vi "Request Live Measurement.vi"(0 "Gas In":refnum<class "Gas.lvclass">, 5 "Request Type":u8=160 format="%x", 11 "error in (no error)":errorcluster) -> (4 "Gas Out":refnum<class "Gas.lvclass">, 6 "Success?":bool, 15 "error out":errorcluster)   [LabVIEW 2015, in "Gas.lvclass"]
uses:
  Gas.lvclass
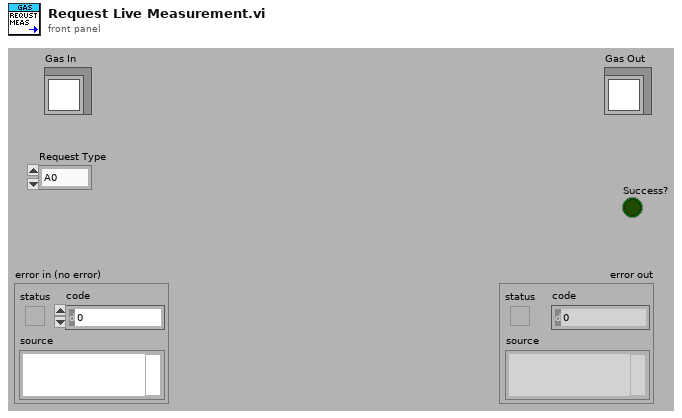
[diagram p1: front panel]
types:
  T1 = typedef "XNET Frame CAN.ctl" = cluster{"timestamp":timestamp, "payload":u8[], "identifier":u32, "type":T2, "extended?":bool, "echo?":bool}
  T2 = typedef "XNET Frame Type CAN.ctl" = u8
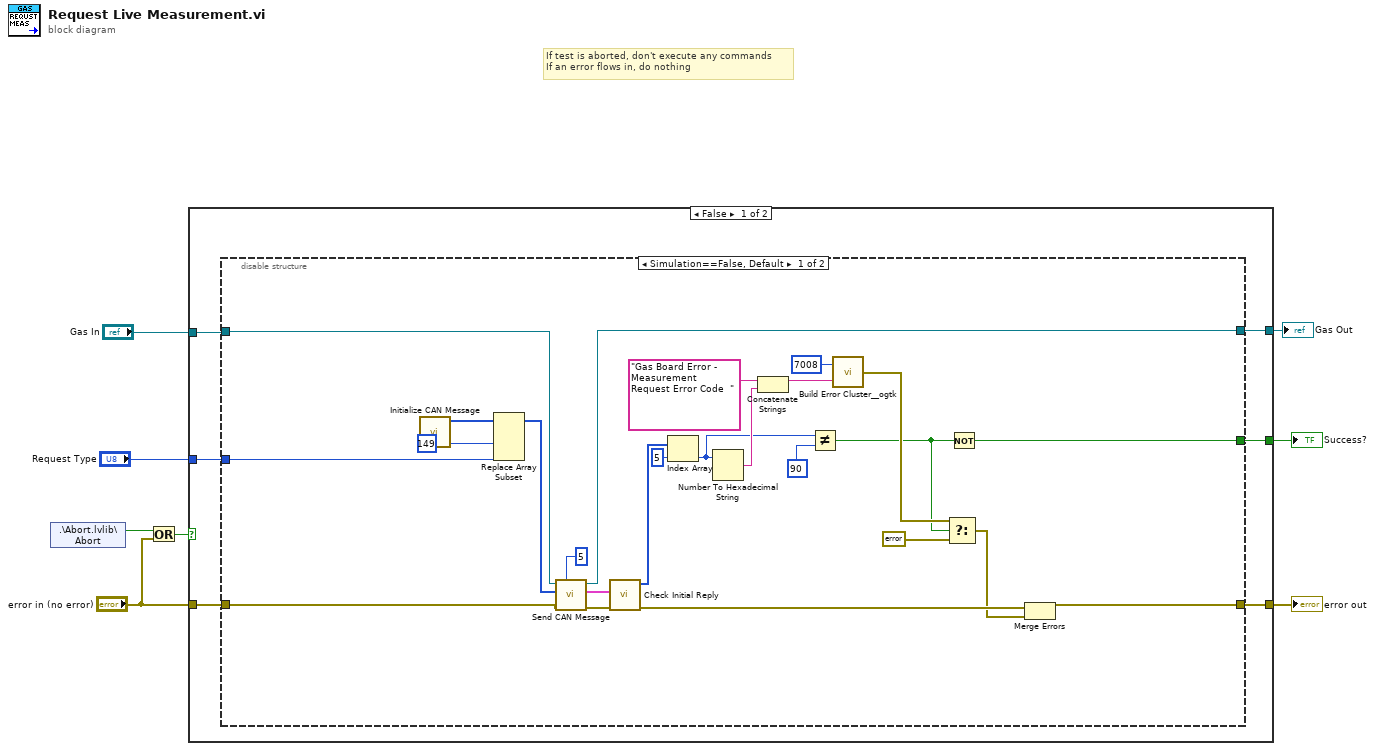
[diagram p0: block diagram]
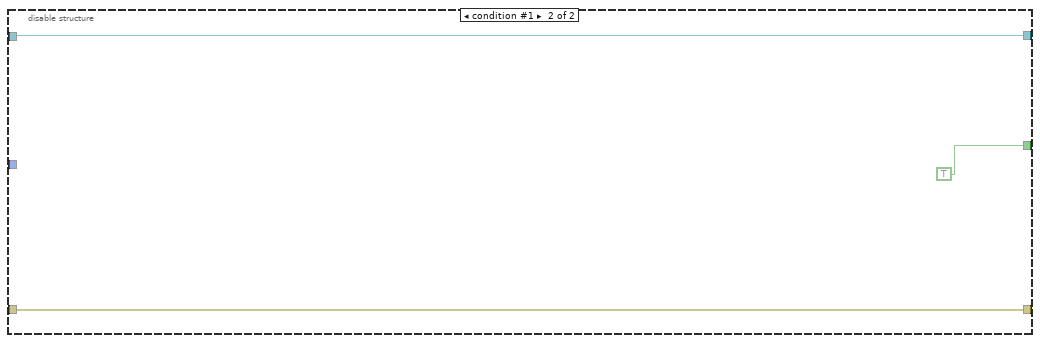
[diagram p2: hidden frame]
diagram:
  # "If test is aborted, don't execute any commands\nIf an error flows in, do nothing"
  n1 = shared-variable ".\\Abort.lvlib\\Abort"() -> (w7:bool)  [unwired: 1 in, 1 out]
  n2 = Or(x=w7, y="error in (no error)") -> (x .or. y?=w5:bool)
  n3 = case shown="False" w5 {
    tunnel: [w14 w44] -> w8
    tunnel: "error in (no error)" -> [w13 w44]
    tunnel: [w12 _] -> w4
    tunnel: "Request Type" -> [w11 _]
    tunnel: "Gas In" -> [w10 w43]
    tunnel: [w9 w43] -> w1
    frame False {
      n4 = disable-structure shown="Simulation==False, Default" {
        disable-tunnel: [w16 w42] -> w14
        disable-tunnel: w10 -> [w21 w40]
        disable-tunnel: w13 -> [w15 w42]
        disable-tunnel: [w39 TRUE] -> w12
        disable-tunnel: w11 -> [w38 _]
        disable-tunnel: [w20 w40] -> w9
        frame condition #0 (active) {
          n5 = call "Initialize CAN Message.vi"() -> ("Initial Payload"=w24:u8[])  [unwired: 11 in]
          n6 = Replace Array Subset(array=w24, new element #1=u8 149 ("new element/subarray"), new element #2=w38) -> (w22:u8[])  [unwired: 2 in]
          n7 = call "Send CAN Message.vi"("Number of Retries"=5, "error in (no error)"=w15, "payload"=w22, "Gas In"=w21) -> ("error out"=w19:errorcluster, "Reply"=w36:T1[], "Gas Out"=w20:refnum<class "Gas.lvclass">)  [unwired: 5 in]
          n8 = call "Check Initial Reply.vi"("error in (no error)"=w19, "Reply"=w36) -> ("error out"=w18:errorcluster, "Data Packet"=w32:u8[])  [unwired: 6 in, 2 out]
          n9 = Index Array(array=w32, index=5) -> (element=w27:u8)
          n10 = Number To Hexadecimal String(2:w27) -> (0:w29:string)  [unwired: 1 in]
          n11 = Concatenate Strings("Gas Board Error -  Measurement Request Error Code  " ("string"), w29) -> (w28:string)
          n12 = Not Equal?(x=w27, y=u8 90 ("new element/subarray")) -> (x != y?=w25:bool)
          n13 = call <userlib>:"Build Error Cluster__ogtk.vi"("String to Prepend to source (\"\")"=w28, "code"=7008) -> ("error out"=w34:errorcluster)
          n14 = Select(t=w34, s=w25, f=errorcluster {"status"=FALSE, "code"=0, "source"=""}) -> (s? t:f=w17:errorcluster)
          n15 = Not(x=w25) -> (.not. x?=w39:bool)
          n16 = Merge Errors(w18, w17) -> (w16:errorcluster)
        }
        frame condition #1 {
        }
      }
    }
    frame True {
    }
  }
  "error out" <- w8
  "Success?" <- w4
  "Gas Out" <- w1
